vi "Send autofocus info.vi"(8 "error in (no error)":errorcluster, 11 "Tomo in":refnum<class "Tomo.lvclass">) -> (0 "error out":errorcluster, 3 "Tomo out":refnum<class "Tomo.lvclass">)   [LabVIEW 2012, in "Tomo.lvclass"]
uses:
  Tomo.lvclass
  <vilib>/Distrio/Murmex/Murmex/update_cluster.ctl
  <vilib>/Distrio/Murmex/Murmex/Murmex.lvclass
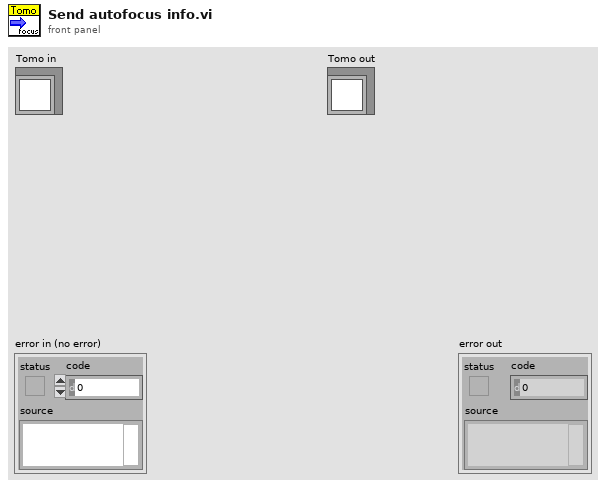
[diagram p1: front panel]
types:
  T1 = typedef "Murmex.lvlib/Murmex.lvclass/update_cluster.ctl" = cluster{"target ID":string, "key chains":string[], "values":variant[]}
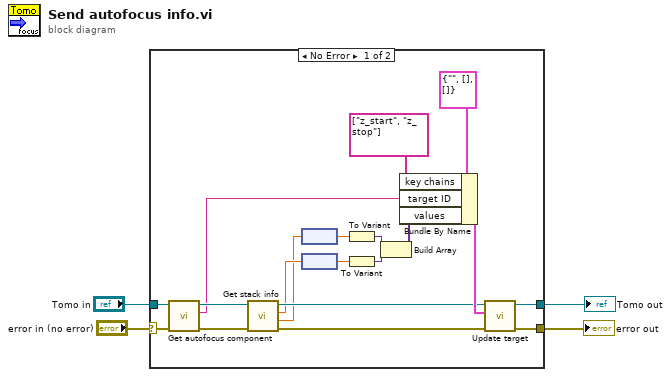
[diagram p0: block diagram]
diagram:
  n1 = case shown="No Error" "error in (no error)" {
    selector: "error in (no error)" -> [w14 w25]
    tunnel: [w18 w25] -> w3
    tunnel: [w20 w24] -> w2
    tunnel: "Tomo in" -> [w16 w24]
    frame No Error {
      n2 = call-dynamic "Get autofocus component.vi"("error in (no error)"=w14, "Tomo in"=w16) -> ("error out"=w13:errorcluster, "autofocus component"=w12:string, "Tomo out"=w15:refnum<class "Tomo.lvclass">)  [unwired: 7 in]
      n3 = call-dynamic "Get stack info.vi"("error in (no error)"=w13, "Tomo in"=w15) -> ("error out"=w19:errorcluster, "Z start"=w10:dbl, "Z stop"=w11:dbl, "Tomo out"=w21:refnum<class "Tomo.lvclass">)  [unwired: 4 in, 2 out]
      n4 = node(w10) -> (w9:dbl[unit])
      n5 = node(w11) -> (w8:dbl[unit])
      n6 = To Variant(anything=w9) -> (Variant=w7:variant)
      n7 = To Variant(anything=w8) -> (Variant=w6:variant)
      n8 = Build Array(w7, w6) -> (w5:variant[])
      n9 = Bundle By Name(cluster=T1 {"target ID"="", "key chains"=[], "values"=[]} ("update cluster"), "key chains"=string[] ["z_start", "z_stop"], "target ID"=w12, "values"=w5) -> (w23:T1)
      n10 = call <vilib>:"Update target.vi"("error in (no error)"=w19, "update cluster"=w23, "MurmexBase in"=w21) -> ("error out"=w18:errorcluster, "MurmexBase out"=w20:refnum<class "Tomo.lvclass">)  [unwired: 7 in]
    }
    frame Error {
    }
  }
  "error out" <- w3
  "Tomo out" <- w2
